vi "ErrorHandlerSIMPLE.vi"() -> (2 "Sorted Timestamps":dbl[](array[numeric]), 3 "Error Cluster Out":T1(array[cluster]))   [LabVIEW 2013]
uses:
  GlobalErrorCAN_ID.vi
  ErrorPrevValues.vi
  GlobalBoardIDs.vi
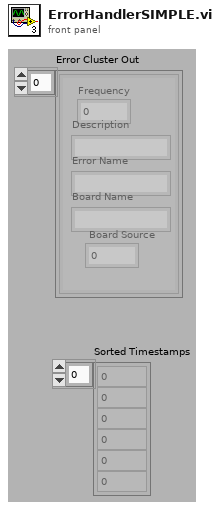
[diagram p1: front panel]
types:
  T1 = cluster{"Frequency":dbl, "Description":string, "Error Name":string, "Board Name":string, " Board Source":dbl}[]
  T2 = cluster{i32, "Description":string, "Error Name":string, "Board Names":string, i32}
  T3 = cluster{i32, "Description":string, "Error Name":string, "Board Names":string, i32}[]
  T4 = cluster{i32, "Description":string, "Error Name":string, "String":string, i32}
  T5 = cluster{i32, "Description":string, "Error Name":string, "String":string, i32}[]
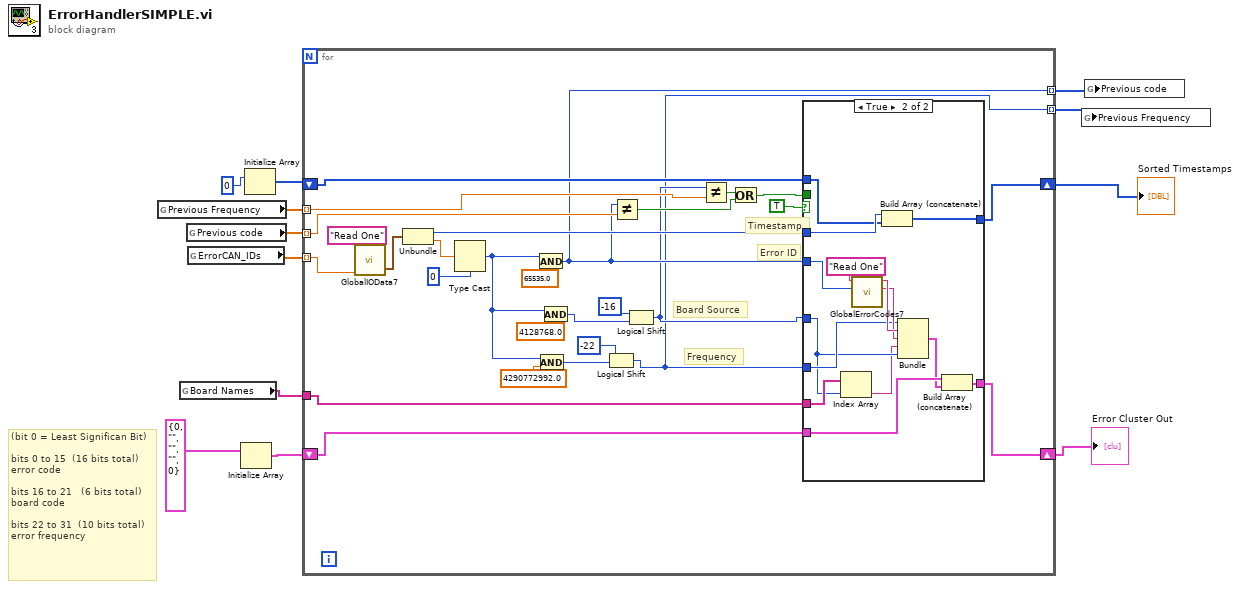
[diagram p0: block diagram]
diagram:
  # "(bit 0 = Least Significan Bit)\n \nbits 0 to 15  (16 bits total)\nerror code\n \nbits 16 to 21   (6 bits total)\nboard code\n \nbits 22 to 31  (10 bits total)\nerror frequency"
  n1 = global read "ErrorPrevValues.vi" "Previous Frequency"() -> (w8:dbl[])
  n2 = global read "GlobalBoardIDs.vi" "Board Names"() -> (w1:string[])
  n3 = global read "ErrorPrevValues.vi" "Previous code"() -> (w7:dbl[])
  n4 = global read "GlobalErrorCAN_ID.vi" "ErrorCAN_IDs"() -> (w9:dbl[])
  n5 = Initialize Array(T2 {0, "Description"="", "Error Name"="", "Board Names"="", 0} ("output cluster")) -> (w12:T3)  [unwired: 1 in]
  n6 = Initialize Array(i8 0 ("y")) -> (w10:i8[])  [unwired: 1 in]
  n7 = for {
    tunnel: w9 -> [w29] mode=indexing
    tunnel: [w24] -> w6 mode=indexing
    tunnel: [w13] -> w5 mode=indexing
    tunnel: w8 -> [w34] mode=indexing
    tunnel: w7 -> [w33] mode=indexing
    shift-right: [w27] -> w3
    shift-left: w12 -> [w28]
    shift-right: [w25] -> w4
    shift-left: w10 -> [w26]
    tunnel: w1 -> [w14]
    # "Timestamp"
    # "Board Source"
    # "Error ID"
    # "Frequency"
    n8 = call "GlobalIOData7.vi"("Function select"="Read One", "IO Data ID"=w29) -> ("IO data out"=w40:cluster{"Time":u32, "Value":sgl})  [unwired: 3 in, 1 out]
    n9 = Unbundle(w40) -> ("Time"=w30:u32, "Value"=w22:sgl)
    n10 = Type Cast(type=u32 0, x=w22) -> (*(type *) &x=w18:u32)
    n11 = And(x=w18, y=sgl 65535.0) -> (x .and. y?=w24:i32)
    n12 = And(x=w18, y=sgl 4290773000.0) -> (x .and. y?=w16:i32)
    n13 = And(x=w18, y=sgl 4128768.0) -> (x .and. y?=w36:i32)
    n14 = Logical Shift(y=i8 -22, x=w16) -> (x << y=w13:i32)
    n15 = Not Equal?(x=w24, y=w33) -> (x != y?=w32:bool)
    n16 = Logical Shift(y=i8 -16, x=w36) -> (x << y=w23:i32)
    n17 = Not Equal?(x=w23, y=w34) -> (x != y?=w31:bool)
    n18 = Or(x=w31, y=w32) -> (x .or. y?=w20:bool)
    n19 = case shown="True" TRUE {
      tunnel: w30 -> [_ w55]
      tunnel: w24 -> [_ w54]
      tunnel: w23 -> [_ w45]
      tunnel: w14 -> [_ w46]
      tunnel: w28 -> [w42 w56]
      tunnel: w26 -> [w41 w51]
      tunnel: [w42 w50] -> w27
      tunnel: [w41 w49] -> w25
      tunnel: w20 -> [_ _]
      tunnel: w13 -> [_ w47]
      frame False {
      }
      frame True {
        n20 = Index Array(array=w46, index=w45) -> (element=w44:string)
        n21 = call "GlobalErrorCodes7.vi"("Element #"=w54, "Function select"="Read One") -> ("Error Name"=w52:string, "Description"=w53:string)  [unwired: 2 in, 2 out]
        n22 = Build Array (concatenate)(w55, w51) -> (w49:u32[])
        n23 = Bundle(w47, "Description"=w53, "Error Name"=w52, "String"=w44, w45) -> (w43:T4)  [unwired: 1 in]
        n24 = Build Array (concatenate)(w56, w43) -> (w50:T5)
      }
    }
  }
  "Error Cluster Out" <- w3
  "Sorted Timestamps" <- w4
  n25 = global write "ErrorPrevValues.vi" "Previous Frequency"(w5) -> ()
  n26 = global write "ErrorPrevValues.vi" "Previous code"(w6) -> ()
